vi "analyseImage.vi"(8 "error in (no error)":errorcluster, 10 "Array":T1(array[cluster]), 11 "AbsorptionDS in":refnum<class "AbsorptionDS.lvclass">) -> (0 "error out":errorcluster, 3 "AbsorptionDS out":refnum<class "AbsorptionDS.lvclass">)   [LabVIEW 2011, in "Tools.lvlib" / "Imaging.lvlib" / "AbsorptionDS.lvclass"]
uses:
  AbsorptionDS.lvclass
  Filing/FileNeologist/FileNeologist.lvclass
  ImageAnalyser.lvclass
  Filing/FileSystem/FileSystem.lvclass
  Imaging.lvlib
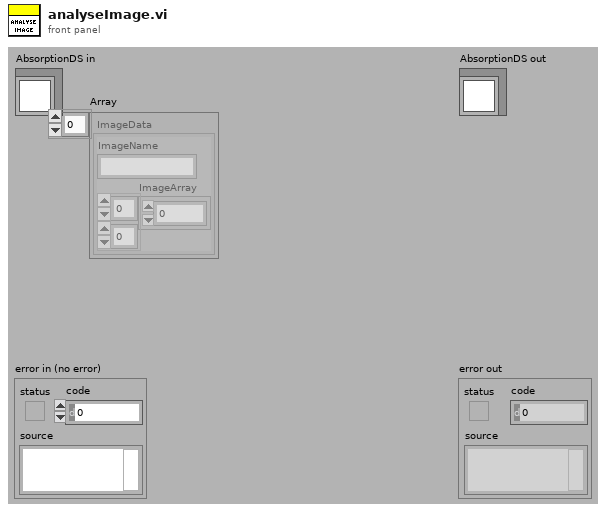
[diagram p1: front panel]
types:
  T1 = cluster{"ImageName":string, "ImageArray":sgl[][]}[]
  T2 = cluster{"Name":string, "Results":dbl[], "AnalysisType":string}
  T3 = cluster{"Left":i32, "Top":i32, "Right":i32, "Bottom":i32}
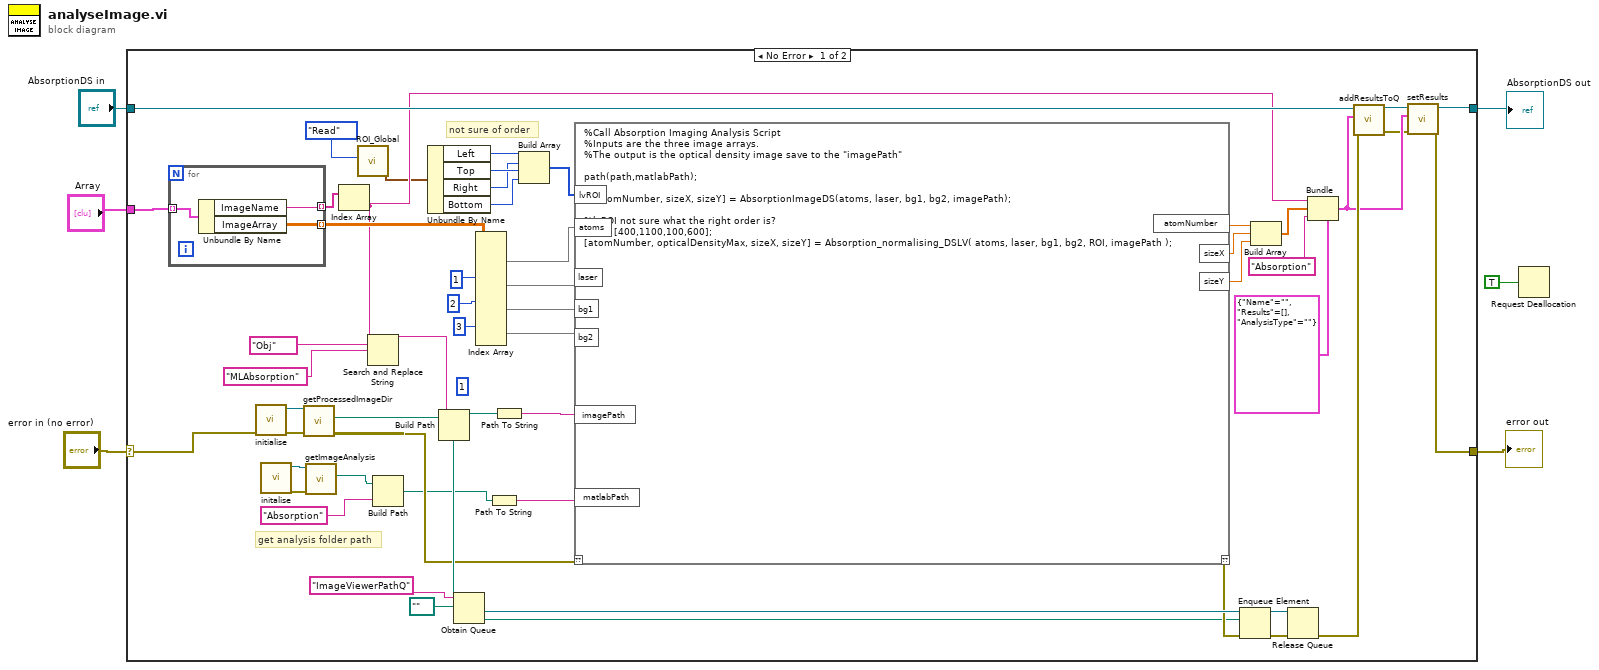
[diagram p0: block diagram]
diagram:
  n1 = case shown="No Error" "error in (no error)" {
    selector: "error in (no error)" -> [w29 w64]
    tunnel: [w17 w64] -> w4
    tunnel: [w20 w63] -> w3
    tunnel: "AbsorptionDS in" -> [w58 w63]
    tunnel: "Array" -> [w57 _]
    frame No Error {
      (unwired) 1
      # "not sure of order"
      # "get analysis folder path"
      n2 = for {
        tunnel: w57 -> [w62] mode=indexing
        tunnel: [w61] -> w56 mode=indexing
        tunnel: [w60] -> w52 mode=indexing
        n3 = Unbundle By Name(w62) -> ("ImageName"=w60:string, "ImageArray"=w61:sgl[][])
      }
      n4 = call "initialise.vi"("error in (no error)"=w29) -> ("error out"=w48:errorcluster, "FileNeologist out"=w49:refnum<class "FileNeologist.lvclass">)  [unwired: 9 in]
      n5 = call "initalise.vi"() -> ("error out"=w25:errorcluster, "FileSystem out"=w26:refnum<class "FileSystem.lvclass">)  [unwired: 10 in]
      n6 = call-dynamic "getProcessedImageDir.vi"("error in (no error)"=w48, "FileNeologist in"=w49) -> ("error out"=w28:errorcluster, "Path"=w47:path)  [unwired: 7 in, 1 out]
      n7 = call "getImageAnalysis.vi"("error in (no error)"=w25, "FileSystem in"=w26) -> ("ImageAnalysis"=w24:path)  [unwired: 7 in, 2 out]
      n8 = Index Array(array=w52) -> (element=w32:string)  [unwired: 1 in]
      n9 = call "ROI_Global.vi"("Action"=enum16{"Write", "Read"}."Read") -> ("ROI"=w12:T3)  [unwired: 10 in]
      n10 = Search and Replace String(input string=w32, search string="Obj", replace string="MLAbsorption") -> (result string=w46:string)  [unwired: 5 in, 3 out]
      n11 = Build Path(base path=w24, name or relative path="Absorption") -> (appended path=w22:path)
      n12 = Unbundle By Name(w12) -> ("Left"=w11:i32, "Top"=w10:i32, "Right"=w9:i32, "Bottom"=w8:i32)
      n13 = Build Path(base path=w47, name or relative path=w46) -> (appended path=w35:path)
      n14 = Obtain Queue(name (unnamed)="ImageViewerPathQ", element data type=path "") -> (queue out=w43:refnum<queue>)  [unwired: 3 in, 2 out]
      n15 = Index Array(array=w56, index (dim 0) #2=1, index (dim 0) #3=2, index (dim 0) #4=3) -> (element #1=w14:sgl[][], element #2=w54:sgl[][], element #3=w53:sgl[][], element #4=w15:sgl[][])  [unwired: 9 in]
      n16 = Path To String(path=w22) -> (string=w27:string)
      n17 = Path To String(path=w35) -> (string=w40:string)
      n18 = Build Array(w11, w9, w10, w8) -> (w7:i32[])
      n19 = script code="%Call Absorption Imaging Analysis Script \n%Inputs are the three image arrays.\n%The output is the optical density image save to the \"imagePath\"\n\npath(path,matlabPath);\n\n%[atomNumber, sizeX, sizeY] = AbsorptionImageDS(atoms, laser, bg1, bg2, imagePath);\n\n%lvROI not sure what the right order is? \nROI = [400,1100,100,600];\n[atomNumber, opticalDensityMax, sizeX, sizeY] = Absorption_normalising_DSLV( atoms, laser, bg1, bg2, ROI, imagePath );"("??"=w28, "bg1"=w53, "laser"=w54, "atoms"=w14, "imagePath"=w40, "matlabPath"=w27, "bg2"=w15, "lvROI"=w7) -> ("??"=w36:errorcluster, "atomNumber"=w39:dbl, "sizeX"=w38:dbl, "sizeY"=w37:dbl)
      n20 = Enqueue Element(queue=w43, element=w35, error in (no error)=w36) -> (queue out=w42:refnum<queue>, error out=w41:errorcluster)  [unwired: 1 in, 1 out]
      n21 = Build Array(w39, w38, w37) -> (w33:dbl[])
      n22 = Release Queue(queue=w42, error in (no error)=w41) -> (error out=w34:errorcluster)  [unwired: 1 in, 2 out]
      n23 = Bundle(cluster=T2 {"Name"="", "Results"=[], "AnalysisType"=""} ("output cluster"), "Name"=w32, "Results"=w33, "AnalysisType"="Absorption") -> (w19:T2)
      n24 = call "addResultsToQ.vi"("error in (no error)"=w34, "Results"=w19, "ImageAnalyser in"=w58) -> ("error out"=w18:errorcluster, "ImageAnalyser out"=w21:refnum<class "AbsorptionDS.lvclass">)  [unwired: 7 in]
      n25 = call "setResults.vi"("error in (no error)"=w18, "results"=w19, "ImageAnalyser in"=w21) -> ("error out"=w17:errorcluster, "ImageAnalyser out"=w20:refnum<class "AbsorptionDS.lvclass">)  [unwired: 7 in]
    }
    frame Error {
    }
  }
  "error out" <- w4
  "AbsorptionDS out" <- w3
  n26 = Request Deallocation(TRUE ("flag")) -> ()
